vi "CSM - Destroy Global Log Event.vi"(8 "Error in":errorcluster caption="Error in (no error)", 11 "JKISM Global Log Event":refnum<user-event>) -> (0 "Error out":errorcluster)   [LabVIEW 2014, in "Communicable State Machine.lvlib"]
doc: "Release CSM Global Log Event Reference.\n\n<b>Inputs:</b>\n - <b>CSM Global Log Event</b>:\n - <b>Error in</b>: Error cluster\n\n<b>Outputs:</b>\n - <b>Error out</b>: Error cluster"
uses:
  Communicable State Machine.lvlib
  _Support/Typedef/_CSM_GlobalLog_MSG.ctl
  _Support/Typedef/_CSM_GlobalLog_MSG_TYPE.ctl
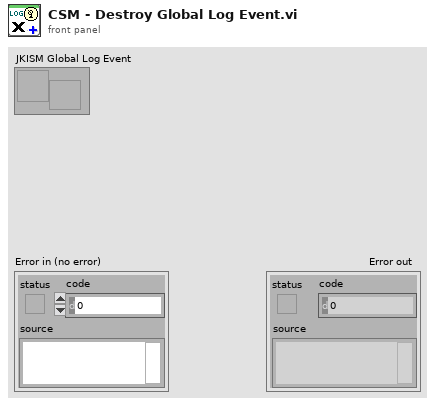
[diagram p1: front panel]
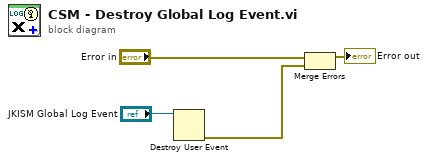
[diagram p0: block diagram]
diagram:
  n1 = Destroy User Event(user event="JKISM Global Log Event") -> (error out=w4:errorcluster)  [unwired: 1 in]
  n2 = Merge Errors("Error in", w4) -> (→"Error out":errorcluster)
